vi "Find_unknown_files.vi"() -> ()   [LabVIEW 2013]
uses:
  <vilib>/addons/database/Connection.llb/Conn Execute.vi
  <vilib>/addons/database/Recordset.llb/Rec Fetch Recordset Data (R).vi
  <vilib>/addons/database/Recordset.llb/Rec Destroy - Connection.vi
  <userlib>/_OpenG.lib/array/array.llb/Conditional Auto-Indexing Tunnel (String)__ogtk.vi
  <userlib>/_OpenG.lib/array/array.llb/Conditional Auto-Indexing Tunnel (I32)__ogtk.vi
  <vilib>/addons/database/_DB Variant To Data/Database Variant To Data.xnode
  <vilib>/addons/database/NI_Database_API.lvlib
panel:
  out "SQL Query":string
  out "Files not Found":string[](array[string])
  out "All File Paths":path[](array[path])
  out "error out":errorcluster
  in  "error in (no error)":errorcluster
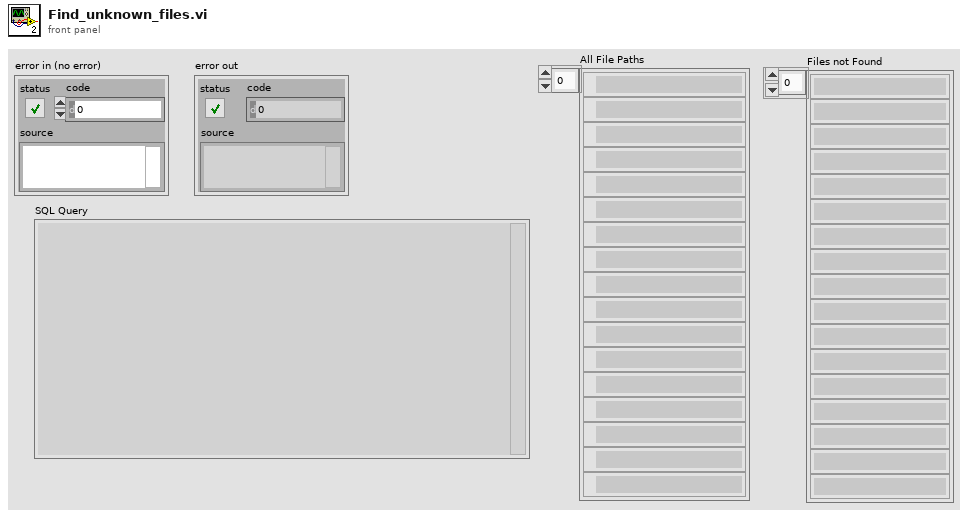
[diagram p1: front panel]
types:
  T1 = typedef "NI_Database_API.lvlib/Conn ObjectReference.ctl" = refnum<k1>
  T2 = typedef "NI_Database_API.lvlib/Rec ObjectReference.ctl" = refnum<k1>
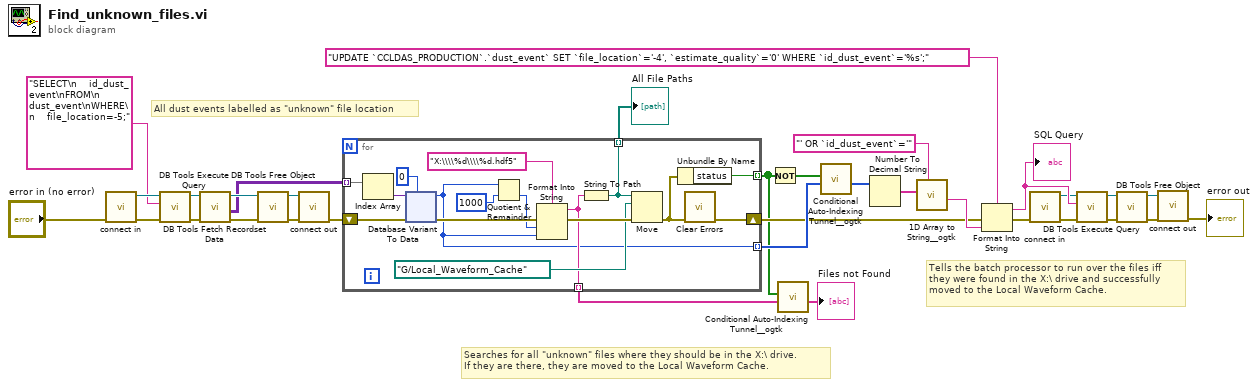
[diagram p0: block diagram]
diagram:
  # "Tells the batch processor to run over the files iff\nthey were found in the X:\\ drive and successfully\nmoved to the Local Waveform Cache."
  # "Searches for all \"unknown\" files where they should be in the X:\\ drive.\nIf they are there, they are moved to the Local Waveform Cache."
  # "All dust events labelled as \"unknown\" file location"
  n1 = call "connect in.vi"("error in (no error)"="error in (no error)") -> ("error out"=w29:errorcluster, "Database Connection"=w28:T1)  [unwired: 6 in, 1 out]
  n2 = call-poly <vilib>:"DB Tools Execute Query.vi"("error in (no error)"=w29, "SQL query"="SELECT\n    id_dust_event\nFROM\n    dust_event\nWHERE\n    file_location=-5;", "connection reference"=w28) -> ("error out"=w30:errorcluster, "recordset reference"=w31:T2)  [unwired: 5 in]
  n3 = call-poly <vilib>:"DB Tools Fetch Recordset Data.vi"("error in (no error)"=w30, "recordset reference"=w31) -> ("error out"=w33:errorcluster, "recordset data"=w23:variant[][], "recordset reference out"=w32:T2)  [unwired: 3 in]
  n4 = call-poly <vilib>:"DB Tools Free Object.vi"("error in (no error)"=w33, "recordset reference"=w32) -> ("error out"=w27:errorcluster, "connection reference"=w26:T1)  [unwired: 8 in]
  n5 = call "connect out.vi"("error in (no error)"=w27, "connection reference"=w26) -> ("error out"=w22:errorcluster)  [unwired: 9 in]
  n6 = for {
    tunnel: w23 -> [w49] mode=indexing
    shift-right: [w41] -> w12
    shift-left: w22 -> [w48]
    tunnel: [w38] -> w21 mode=indexing
    tunnel: [w37] -> w7 mode=indexing
    tunnel: [w36] -> w20 mode=indexing
    tunnel: [w35] -> w18 mode=indexing
    n7 = Index Array(array=w49) -> (element=w47:variant)  [unwired: 1 in]
    n8 = xnode "Database Variant To Data"("database variant"=w47, "error in (no error)"=w48, "type"=0) -> ("data"=w35:i32, "error out"=w44:errorcluster)
    n9 = Quotient & Remainder(x=w35, y=1000 ("data")) -> (floor(x/y)=w42:i32)  [unwired: 1 out]
    n10 = Format Into String(format string="X:\\\\%d\\\\%d.hdf5", error in=w44, w42, w35) -> (resulting string=w36:string, error out=w40:errorcluster)  [unwired: 1 in]
    n11 = String To Path(string=w36) -> (path=w38:path)
    n12 = Move(source path=w38, error in=w40, 10:path "G:/Local_Waveform_Cache") -> (error out=w34:errorcluster)  [unwired: 2 in, 2 out]
    n13 = Unbundle By Name(w34) -> ("status"=w37:bool)
    n14 = call <vilib>:"Clear Errors.vi"("error in (no error)"=w34) -> ("error out"=w41:errorcluster)  [unwired: 6 in]
  }
  "All File Paths" <- w21
  n15 = Not(x=w7) -> (.not. x?=w8:bool[])
  n16 = call-poly <userlib>:"Conditional Auto-Indexing Tunnel__ogtk.vi"("Array in"=w20, "Elements to keep"=w7) -> ("Filtered Array out"=→"Files not Found":string[])  [unwired: 5 in]
  n17 = call-poly <userlib>:"Conditional Auto-Indexing Tunnel__ogtk.vi"("Array in"=w18, "Elements to keep"=w8) -> ("Filtered Array out"=w17:i32[])  [unwired: 5 in]
  n18 = Number To Decimal String(number=w17) -> (decimal integer string=w16:string[])  [unwired: 1 in]
  n19 = call <userlib>:"1D Array to String__ogtk.vi"("delimiter (Tab)"="' OR `id_dust_event`='", "Array of Strings"=w16) -> ("delimited string"=w13:string)  [unwired: 9 in]
  n20 = Format Into String(format string="UPDATE `CCLDAS_PRODUCTION`.`dust_event` SET `file_location`='-4', `estimate_quality`='0' WHERE `id_dust_event`='%s';" ("string"), error in=w12, w13) -> (resulting string=w15:string, error out=w14:errorcluster)  [unwired: 1 in]
  "SQL Query" <- w15
  n21 = call "connect in.vi"("error in (no error)"=w14) -> ("error out"=w4:errorcluster, "Database Connection"=w3:T1)  [unwired: 6 in, 1 out]
  n22 = call-poly <vilib>:"DB Tools Execute Query.vi"("error in (no error)"=w4, "SQL query"=w15, "connection reference"=w3) -> ("error out"=w6:errorcluster, "recordset reference"=w5:T2)  [unwired: 5 in]
  n23 = call-poly <vilib>:"DB Tools Free Object.vi"("error in (no error)"=w6, "recordset reference"=w5) -> ("error out"=w2:errorcluster, "connection reference"=w1:T1)  [unwired: 8 in]
  n24 = call "connect out.vi"("error in (no error)"=w2, "connection reference"=w1) -> ("error out"=→"error out":errorcluster)  [unwired: 9 in]
